vi "Actor Core.vi"(8 "error in":errorcluster, 11 "Side Menu View in":refnum<class "Side Menu View.lvclass">) -> (0 "error out":errorcluster, 3 "Actor out":refnum<class "Actor.lvclass">)   [LabVIEW 2020, in "Side Menu View.lvlib" / "Side Menu View.lvclass"]
doc: "(<B>Filename</B>: Actor Framework.lvlib:Actor.lvclass:Actor Core.vi)\n\nReceives messages to the actor, reacts to them, and initiates any error handling that may shut the actor down.\n\nDescendant classes may override this VI to append parallel tasks for the actor to complete while it handles messages. Overrides use the Call Parent Method node."
uses:
  Side Menu View.lvclass
  C:/Program Files/National Instruments/LabVIEW 2020/vi.lib/ActorFramework/Actor/Actor.lvclass
  <vilib>/ActorFramework/Actor/Actor.lvclass
  Side Menu View.lvclass/Side Menu View.ctl
  <vilib>/ActorFramework/Actor/Actor.lvclass/Actor.ctl
  <vilib>/ActorFramework/Message Enqueuer/Message Enqueuer.lvclass/Message Enqueuer.ctl
  Side Menu View Messages/Broadcast Side Menu Pressed Msg/Broadcast Side Menu Pressed Msg.lvclass/Broadcast Side Menu Pressed Msg.ctl
  Side Menu View Messages/Broadcast Load Pressed Msg/Broadcast Load Pressed Msg.lvclass/Broadcast Load Pressed Msg.ctl
  Side Menu View Messages/Broadcast Save Pressed Msg/Broadcast Save Pressed Msg.lvclass/Broadcast Save Pressed Msg.ctl
  Side Menu View Messages/Broadcast Save As Pressed Msg/Broadcast Save As Pressed Msg.lvclass/Broadcast Save As Pressed Msg.ctl
  Side Menu View Messages/Broadcast About Pressed Msg/Broadcast About Pressed Msg.lvclass/Broadcast About Pressed Msg.ctl
  Side Menu View Messages/Broadcast Settings Pressed Msg/Broadcast Settings Pressed Msg.lvclass/Broadcast Settings Pressed Msg.ctl
  <vilib>/ActorFramework/Message Enqueuer/Init from Existing Queue.vi
  <vilib>/ActorFramework/Message Enqueuer/Enqueue.vi
  Side Menu View Messages/Broadcast Side Menu Pressed Msg/Broadcast Side Menu Pressed Msg.lvclass
  C:/Program Files/National Instruments/LabVIEW 2020/vi.lib/ActorFramework/Message/Message.lvclass
  Side Menu View Messages/Broadcast Load Pressed Msg/Broadcast Load Pressed Msg.lvclass
  Controllers/UI Controller/UI Controller Messages/Initialize Main View Msg/Initialize Main View Msg.lvclass
  Side Menu View Messages/Broadcast Save Pressed Msg/Broadcast Save Pressed Msg.lvclass
  Side Menu View Messages/Broadcast Save As Pressed Msg/Broadcast Save As Pressed Msg.lvclass
  Side Menu View Messages/Broadcast About Pressed Msg/Broadcast About Pressed Msg.lvclass
  Side Menu View Messages/Broadcast Settings Pressed Msg/Broadcast Settings Pressed Msg.lvclass
  <vilib>/ActorFramework/Message Priority Queue/Priority Enqueue.vi
  <vilib>/ActorFrameworkMVC/Abstract View/Abstract View/Abstract View.lvclass
  <vilib>/ActorFramework/Message Enqueuer/Message Enqueuer.lvclass
panel:
  in  "Disabled About Button":bool
  in  "Disabled Save As Button":bool
  in  "Disabled Save Button":bool
  in  "About Button":bool
  in  "Save As Button":bool
  in  "Save Button":bool
  in  "Load Button":bool
  in  "Side Menu Button":bool
  in  "Settings Button":bool
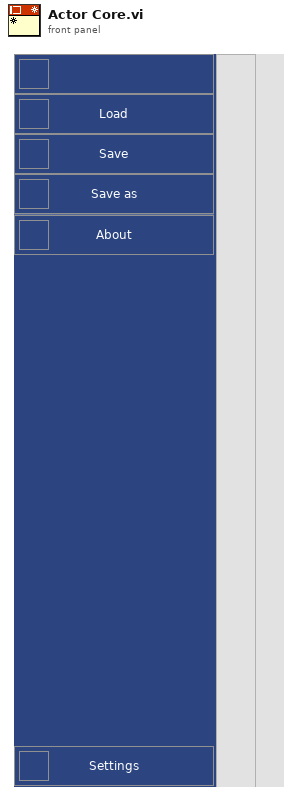
[diagram p1: front panel]
types:
  T1 = enum8{"Enabled", "Disabled", "Disabled and Grayed Out"}
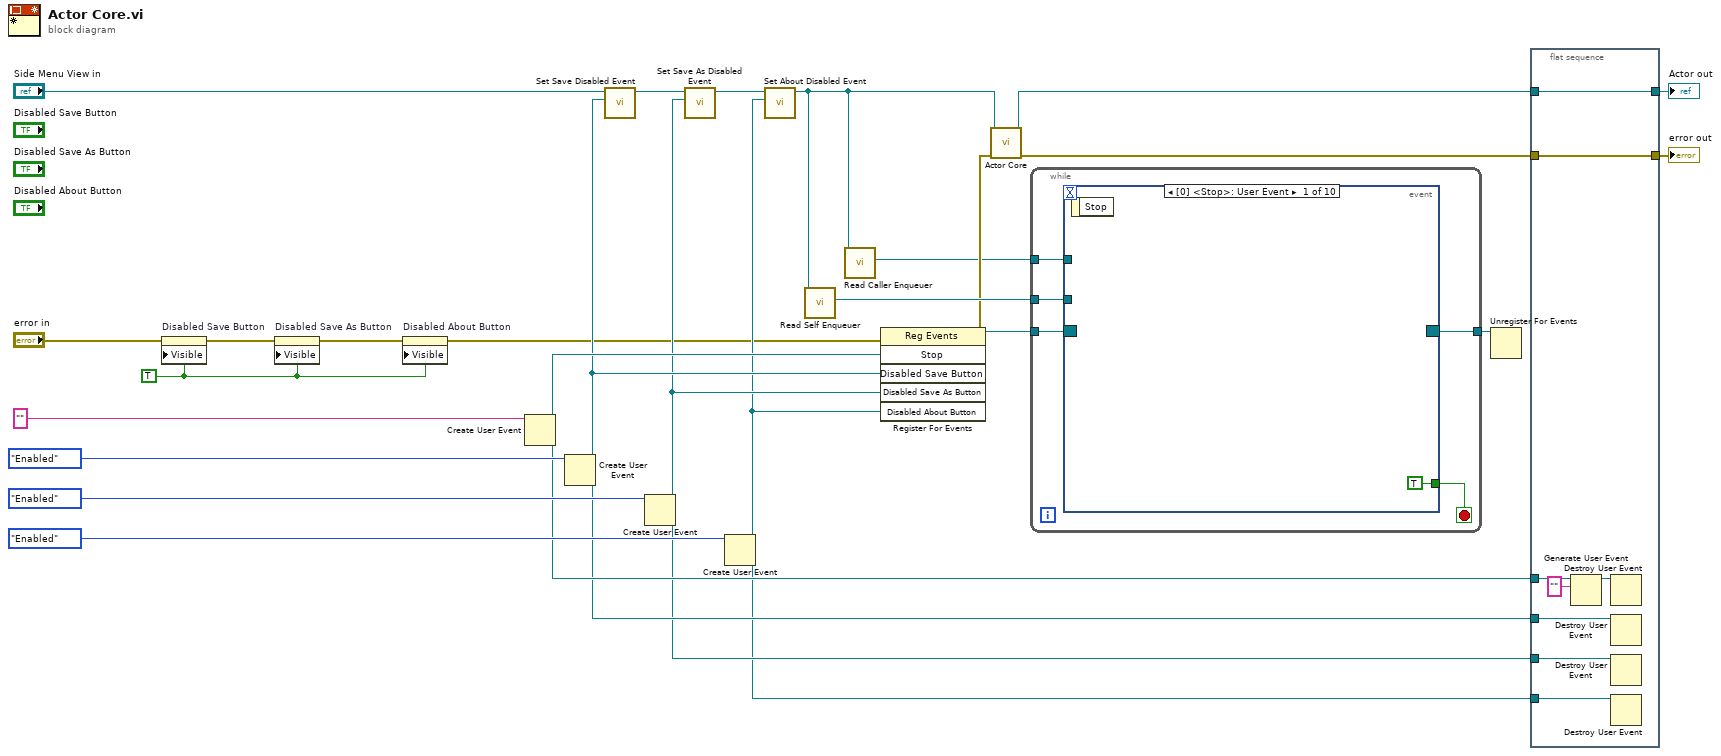
[diagram p0: block diagram]
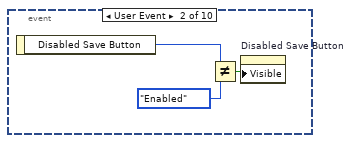
[diagram p2: hidden frame]
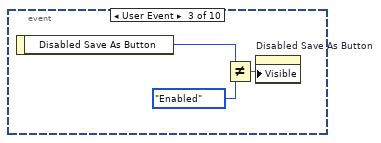
[diagram p3: hidden frame]
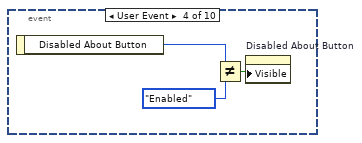
[diagram p4: hidden frame]
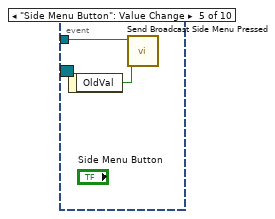
[diagram p5: hidden frame]
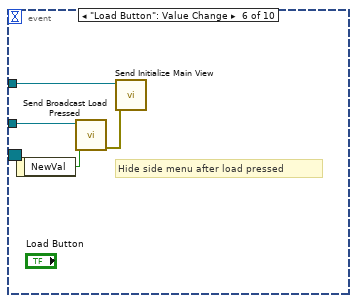
[diagram p6: hidden frame]
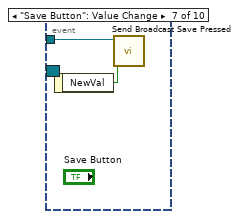
[diagram p7: hidden frame]
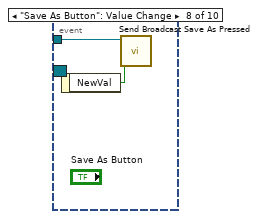
[diagram p8: hidden frame]
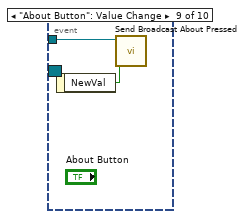
[diagram p9: hidden frame]
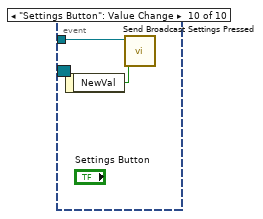
[diagram p10: hidden frame]
diagram:
  w4 = TRUE ("Visible")
  n1 = property on="Disabled Save Button" class="Bool"(error in="error in", "Visible"=w4) -> (error out=w7:errorcluster)  [unwired: 1 in, 1 out]
  n2 = property on="Disabled Save As Button" class="Bool"(error in=w7, "Visible"=w4) -> (error out=w6:errorcluster)  [unwired: 1 in, 1 out]
  n3 = property on="Disabled About Button" class="Bool"(error in=w6, "Visible"=w4) -> (error out=w3:errorcluster)  [unwired: 1 in, 1 out]
  n4 = Create User Event(user event datatype="" ("Stop")) -> (user event=w14:refnum<user-event>)  [unwired: 1 in, 1 out]
  n5 = Create User Event(user event datatype=T1."Enabled" ("Disabled Save Button")) -> (user event=w11:refnum<user-event>)  [unwired: 1 in, 1 out]
  n6 = call "Set Save Disabled Event.vi"("Save Disabled Event"=w11, "Side Menu View in"="Side Menu View in") -> ("Side Menu View out"=w13:refnum<class "Side Menu View.lvclass">)  [unwired: 9 in]
  n7 = Create User Event(user event datatype=T1."Enabled" ("Disabled Save As Button")) -> (user event=w10:refnum<user-event>)  [unwired: 1 in, 1 out]
  n8 = call "Set Save As Disabled Event.vi"("Save As Disabled Event"=w10, "Side Menu View in"=w13) -> ("Side Menu View out"=w12:refnum<class "Side Menu View.lvclass">)  [unwired: 9 in]
  n9 = Create User Event(user event datatype=T1."Enabled" ("Disabled About Button")) -> (user event=w9:refnum<user-event>)  [unwired: 1 in, 1 out]
  n10 = call "Set About Disabled Event.vi"("About Disabled Event"=w9, "Side Menu View in"=w12) -> ("Side Menu View out"=w2:refnum<class "Side Menu View.lvclass">)  [unwired: 9 in]
  n11 = call <vilib>:"Read Self Enqueuer.vi"("Actor"=w2) -> ("Self Enqueuer"=w16:refnum<class "Message Enqueuer.lvclass">)  [unwired: 10 in]
  n12 = call <vilib>:"Read Caller Enqueuer.vi"("Actor"=w2) -> ("Caller Enqueuer"=w1:refnum<class "Message Enqueuer.lvclass">)  [unwired: 10 in]
  n13 = register-events(error in=w3, w14, w11, w10, w9) -> (reference out=w22:refnum<event-registration>, error out=w8:errorcluster)  [unwired: 1 in]
  n14 = call-parent "Actor Core.vi"("error in"=w8, "Abstract View in"=w2) -> ("error out"=w19:errorcluster, "Actor out"=w20:refnum<class "Actor.lvclass">)  [unwired: 8 in]
  n15 = while {
    tunnel: w22 -> [w31]
    tunnel: [w30] -> w23
    tunnel: w16 -> [w28]
    tunnel: w1 -> [w27]
    stop <- w29 stop-if-true
    n16 = event shown="[0] <Stop>: User Event" {
      selector: w31 -> [_ _ _ _ _ _ _ _ _ _]
      dyn-events: [_ _ _ _ _ _ _ _ _ _] -> w30
      timeout: _ -> [_ _ _ _ _ _ _ _ _ _]
      tunnel: [TRUE _ _ _ _ _ _ _ _ _] -> w29
      tunnel: w28 -> [_ _ _ _ w43 w47 w49 w51 w53 w55]
      tunnel: w27 -> [_ _ _ _ _ w45 _ _ _ _]
      event User Event {
        n17 = event-data() -> ()  [unwired: 1 in, 1 out]
      }
      event User Event {
        n18 = event-data() -> ("Disabled Save Button"=w35:T1)  [unwired: 1 in]
        n19 = Not Equal?(x=w35, y=T1."Enabled") -> (x != y?=w33:bool)
        n20 = property on="Disabled Save Button" class="Bool"("Visible"=w33) -> ()  [unwired: 2 in, 2 out]
      }
      event User Event {
        n21 = event-data() -> ("Disabled Save As Button"=w38:T1)  [unwired: 1 in]
        n22 = Not Equal?(x=w38, y=T1."Enabled") -> (x != y?=w36:bool)
        n23 = property on="Disabled Save As Button" class="Bool"("Visible"=w36) -> ()  [unwired: 2 in, 2 out]
      }
      event User Event {
        n24 = event-data() -> ("Disabled About Button"=w41:T1)  [unwired: 1 in]
        n25 = Not Equal?(x=w41, y=T1."Enabled") -> (x != y?=w39:bool)
        n26 = property on="Disabled About Button" class="Bool"("Visible"=w39) -> ()  [unwired: 2 in, 2 out]
      }
      event "Side Menu Button": Value Change {
        n27 = event-data() -> ("OldVal"=w42:bool)  [unwired: 1 in]
        n28 = call "Send Broadcast Side Menu Pressed.vi"("Side Menu Pressed"=w42, "Message Enqueuer"=w43) -> ()  [unwired: 8 in, 2 out]
      }
      event "Load Button": Value Change {
        # "Hide side menu after load pressed"
        n29 = event-data() -> ("NewVal"=w46:bool)  [unwired: 1 in]
        n30 = call "Send Broadcast Load Pressed.vi"("Load Pressed"=w46, "Message Enqueuer"=w47) -> ("error out"=w44:errorcluster)  [unwired: 8 in, 1 out]
        n31 = call "Send Initialize Main View.vi"("error in (no error)"=w44, "Message Enqueuer"=w45) -> ()  [unwired: 8 in, 2 out]
      }
      event "Save Button": Value Change {
        n32 = event-data() -> ("NewVal"=w48:bool)  [unwired: 1 in]
        n33 = call "Send Broadcast Save Pressed.vi"("Save Pressed"=w48, "Message Enqueuer"=w49) -> ()  [unwired: 8 in, 2 out]
      }
      event "Save As Button": Value Change {
        n34 = event-data() -> ("NewVal"=w50:bool)  [unwired: 1 in]
        n35 = call "Send Broadcast Save As Pressed.vi"("Save As Pressed"=w50, "Message Enqueuer"=w51) -> ()  [unwired: 8 in, 2 out]
      }
      event "About Button": Value Change {
        n36 = event-data() -> ("NewVal"=w52:bool)  [unwired: 1 in]
        n37 = call "Send Broadcast About Pressed.vi"("About Pressed"=w52, "Message Enqueuer"=w53) -> ()  [unwired: 8 in, 2 out]
      }
      event "Settings Button": Value Change {
        n38 = event-data() -> ("NewVal"=w54:bool)  [unwired: 1 in]
        n39 = call "Send Broadcast Settings Pressed.vi"("Settings Pressed"=w54, "Message Enqueuer"=w55) -> ()  [unwired: 8 in, 2 out]
      }
    }
  }
  n40 = Unregister For Events(event registration refnum=w23) -> ()  [unwired: 1 in, 1 out]
  n41 = flat-sequence {
    tunnel: w14 -> [w62]
    tunnel: w11 -> [w60]
    tunnel: w10 -> [w59]
    tunnel: w20 -> [w58]
    tunnel: [w58] -> w21
    tunnel: [w57] -> w18
    tunnel: w19 -> [w57]
    tunnel: w9 -> [w56]
    frame #0 {
      n42 = Generate User Event(user event=w62, event data cluster="" ("event data")) -> (user event out=w63:refnum<user-event>)  [unwired: 2 in, 1 out]
      n43 = Destroy User Event(user event=w63) -> ()  [unwired: 1 in, 1 out]
      n44 = Destroy User Event(user event=w60) -> ()  [unwired: 1 in, 1 out]
      n45 = Destroy User Event(user event=w59) -> ()  [unwired: 1 in, 1 out]
      n46 = Destroy User Event(user event=w56) -> ()  [unwired: 1 in, 1 out]
    }
  }
  "error out" <- w18
  "Actor out" <- w21
